vi "fp button handler_crMD.vi"(5 "dummy error input (just for timing purposes)":errorcluster) -> ()   [LabVIEW 2012]
doc: "SciScan 1.2 160622"
uses:
  <vilib>/Utility/VariantDataType/Type.ctl
  GFG/GFGallGet.vi
  GFG/GFGfpRefGet.vi
  GFG/GFG library.lvlib
  <vilib>/Utility/VariantDataType/VariantType.lvlib
panel:
  out "Source VI":string
  in  "stop":bool
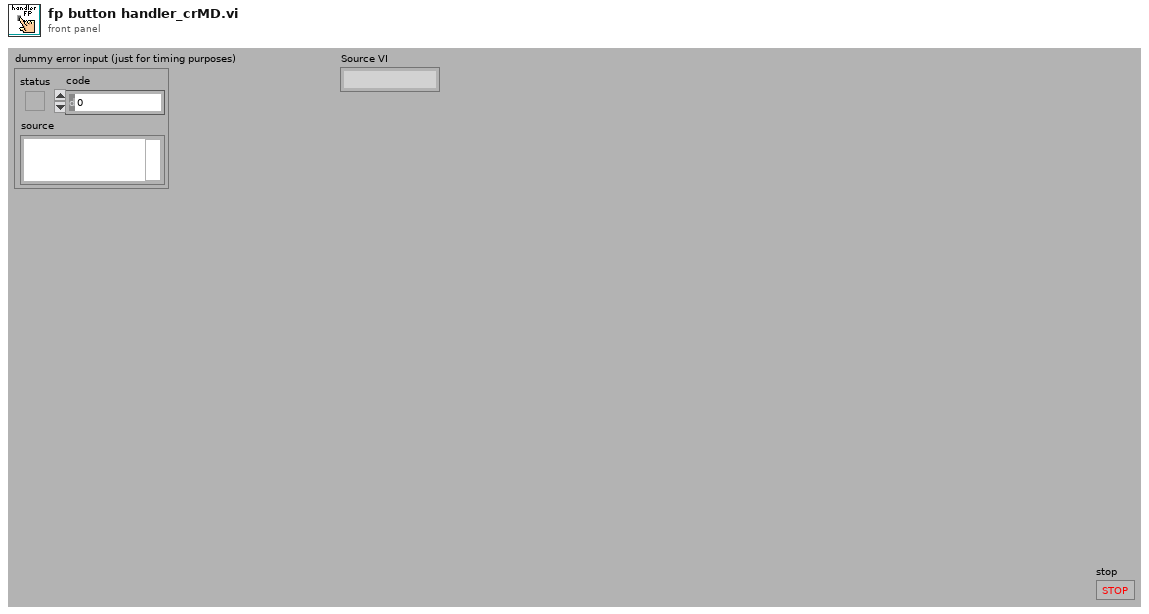
[diagram p1: front panel]
types:
  T1 = enum32{"invalid OS target", "Mac OS", "Windows 3.1", "Windows 95/NT", "Solaris 1", "Solaris 2", "HP-UX", "PowerMAX", "Linux", "Irix", "Rhapsody", "BeOS", "AIX", "OSF1", "VxWorks", "PharLap", "Carbon", "RTX", "Windows x64", "Linux x64"}
  T2 = typedef "VariantType.lvlib/Type.ctl" = enum8{"Invalid Type", "Void", "I8", "I16", "I32", "I64", "U8", "U16", "U32", "U64", "Single Float", "Double Float", "Extended Float", "Single Complex", "Double Complex", "Extended Complex", "Enum U8", "Enum U16", "Enum U32", "Enum U64", "Single Float With Unit", "Double Float With Unit", "Extended Float With Unit", "Single Complex with Unit", "Double Complex with Unit", "Extended Complex with Unit", "Boolean", "String", "Path", "Picture", "Tag", "Array", "Cluster", "Variant", "LV Variant", "Waveform", "Timestamp", "Digital Waveform", "Digital Data", "ExpressData", "Refnum", "External Data", "VI", "Poly VI", "LabVIEW Class Instance", "Fixed Point"}
  T3 = cluster{"Variable Name Out":string, "Data Type Out":T2, "Variant Out":variant}[]
  T4 = cluster{"WaveformChartRef":refnum<vi>, "DigitalRef":refnum<vi>, "ArrayRef":refnum<vi>, "TabControlRef":refnum<vi>, "EnumRef":refnum<vi>, "RingRef":refnum<vi>, "BooleanRef":refnum<vi>, "KnobRef":refnum<vi>, "SlideRef":refnum<vi>, "PathRef":refnum<vi>, "StringRef":refnum<vi>, "ComboBox":refnum<vi>, "WaveformGraphRef":refnum<vi>}
  T5 = enum8{"Enabled", "Disabled", "Disabled and Grayed Out"}
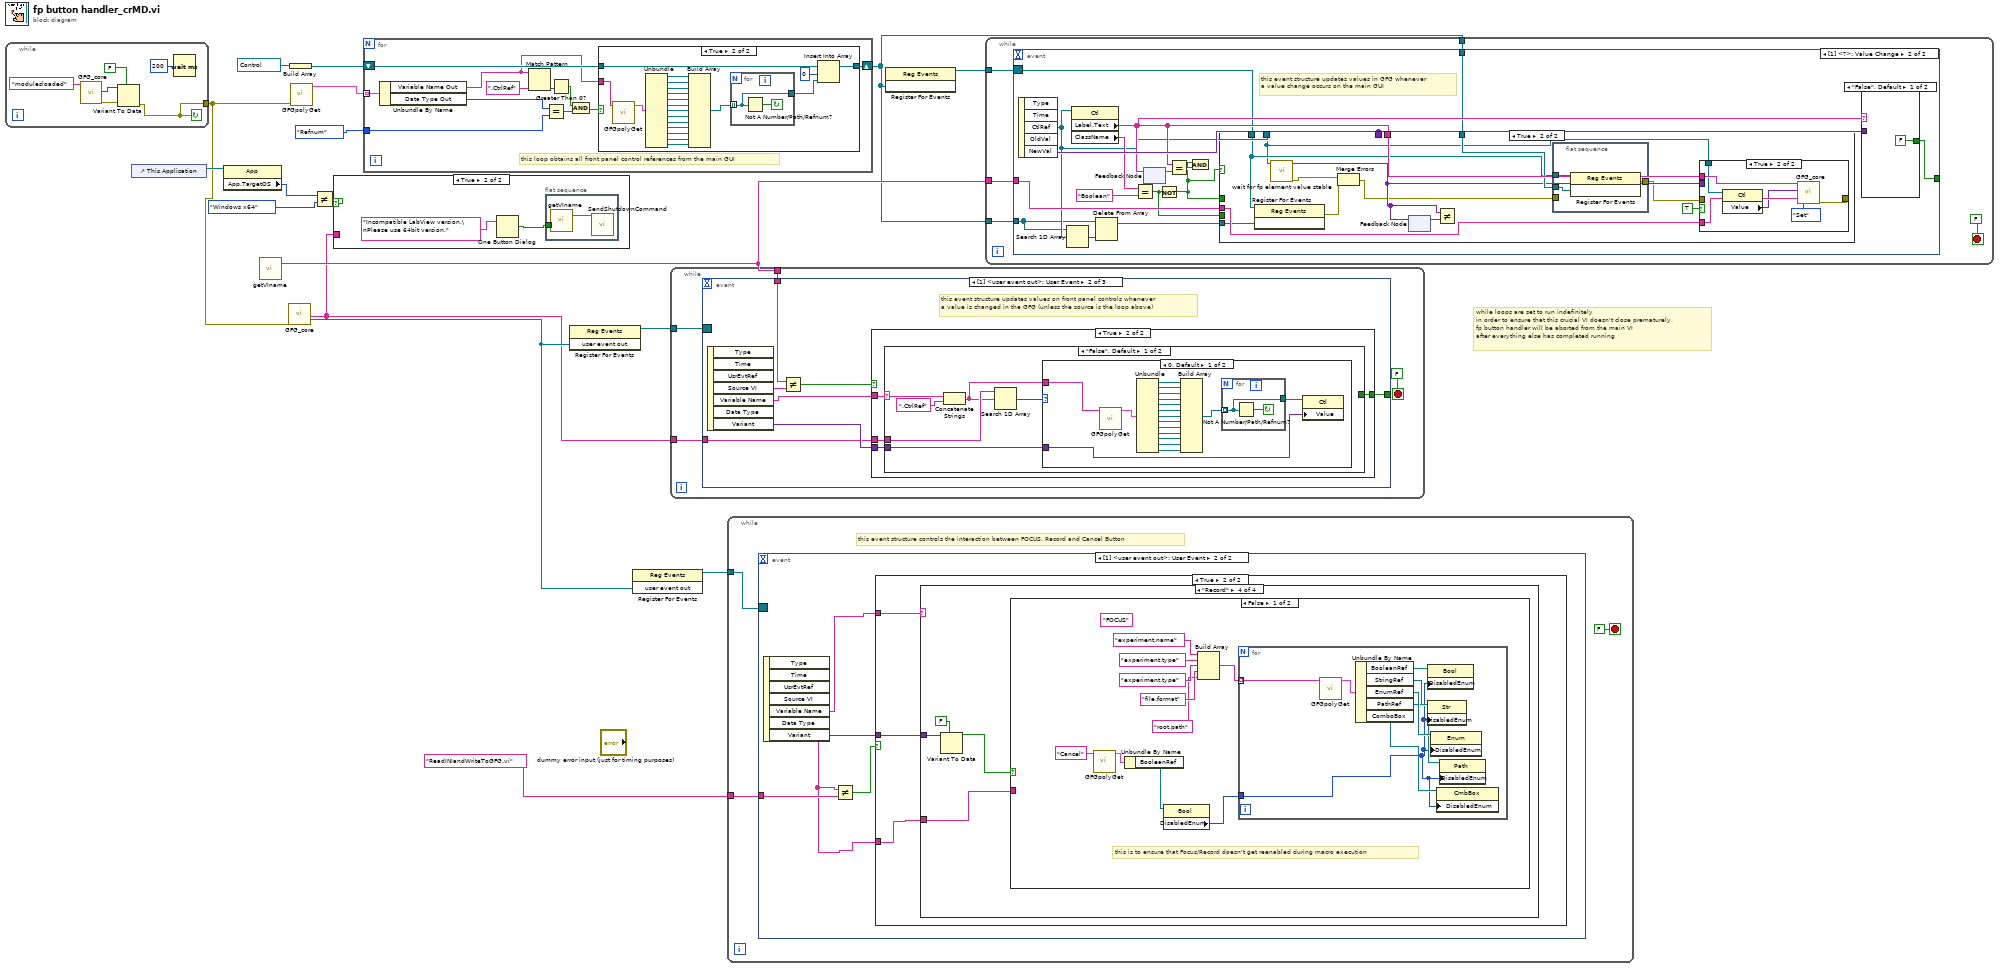
[diagram p0: block diagram]
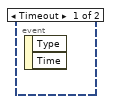
[diagram p3: hidden frame]
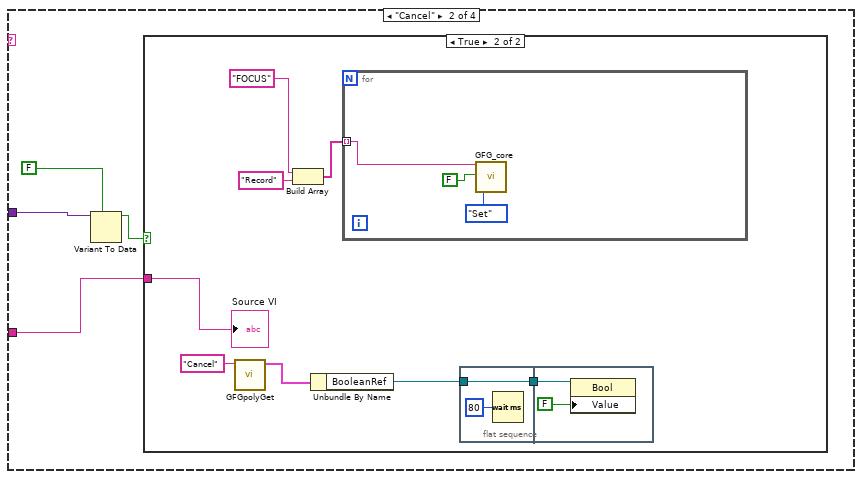
[diagram p6: hidden frame]
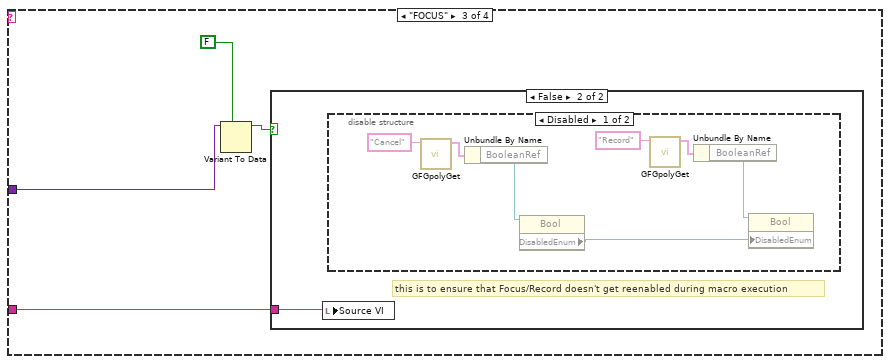
[diagram p8: hidden frame]
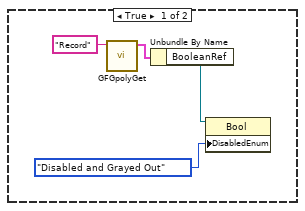
[diagram p9: hidden frame]
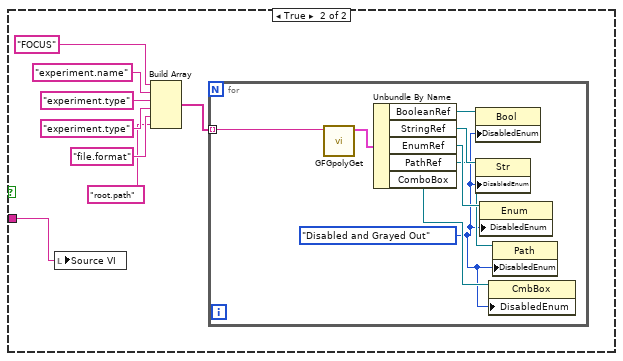
[diagram p11: hidden frame]
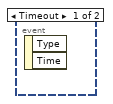
[diagram p12: hidden frame]
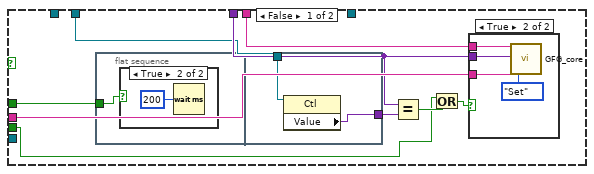
[diagram p13: hidden frame]
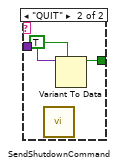
[diagram p17: hidden frame]
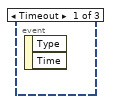
[diagram p19: hidden frame]
diagram:
  # "while loops are set to run indefinitely\nin order to ensure that this crucial VI doesn't close prematurely.\nfp button handler will be aborted from the main VI \nafter everything else has completed running"
  n1 = while {
    tunnel: [w18] -> w2
    stop <- w18 continue-if-true
    n2 = call "GFG_core.vi"("Variable Name in"="modulesloaded") -> ("Variant Out"=w19:variant, "error out"=w21:errorcluster)  [unwired: 12 in, 5 out]
    n3 = Variant To Data(error in=w21, type=FALSE, Variant=w19) -> (error out=w18:errorcluster)  [unwired: 1 out]
    n4 = Wait (ms)(milliseconds to wait=u32 200) -> ()  [unwired: 1 out]
  }
  n5 = control-ref of="This Application"() -> (w7:refnum<vi>)
  n6 = property class="App"(reference=w7) -> ("App.TargetOS"=w6:T1)  [unwired: 1 in, 2 out]
  n7 = call "getVIname.vi"() -> ("VI name"=w11:string)  [unwired: 19 in]
  n8 = call "GFG_core.vi"("error in (no error)"=w2) -> ("All Variable Names Out"=w3:string[], "user event out"=w9:refnum<user-event>)  [unwired: 12 in, 5 out]
  n9 = Build Array(refnum<vi> refnum ("DigitalRef")) -> (w14:refnum<vi>[])
  n10 = call-poly "GFGpolyGet.vi"("error in (no error)"=w2) -> ("Array of Clusters of Variables"=w16:T3)  [unwired: 9 in, 1 out]
  n11 = Not Equal?(x=w6, y=T1."Windows x64" ("Application:Target:Operating System")) -> (x != y?=w4:bool)
  n12 = case shown="True" w4 {
    tunnel: w3 -> [_ _]
    frame False {
    }
    frame True {
      n13 = One Button Dialog(message="Incompatible LabView version.\nPlease use 64bit version." ("source")) -> (true=w24:bool)  [unwired: 1 in]
      n14 = flat-sequence {
        tunnel: w24 -> [_]
        frame #0 {
          n15 = call "getVIname.vi"() -> ("VI name"=w26:string)  [unwired: 19 in]
          n16 = call "SendShutdownCommand.vi"("Source VI"=w26) -> ()  [unwired: 11 in]
        }
      }
    }
  }
  n17 = for {
    tunnel: w16 -> [w37] mode=indexing
    tunnel: Type."Refnum" ("Data Type Out") -> [w35]
    shift-right: [w33] -> w1
    shift-left: w14 -> [w34]
    # "this loop obtains all front panel control references from the main GUI"
    n18 = Unbundle By Name(w37) -> ("Variable Name Out"=w27:string, "Data Type Out"=w36:T2)
    n19 = Match Pattern(string=w27, regular expression=".CtrlRef" ("string")) -> (offset past match=w31:i32)  [unwired: 1 in, 3 out]
    n20 = Equal?(x=w36, y=w35) -> (x = y?=w28:bool)
    n21 = Greater Than 0?(x=w31) -> (x > 0?=w29:bool)
    n22 = And(x=w29, y=w28) -> (x .and. y?=w30:bool)
    n23 = case shown="True" w30 {
      tunnel: w34 -> [w38 w44]
      tunnel: [w38 w43] -> w33
      tunnel: w27 -> [_ w41]
      frame False {
      }
      frame True {
        n24 = call-poly "GFGpolyGet.vi"("Variable Name in"=w41) -> ("output cluster"=w46:T4)  [unwired: 9 in, 1 out]
        n25 = Unbundle(w46) -> ("WaveformChartRef"=w47:refnum<vi>, "DigitalRef"=w48:refnum<vi>, "ArrayRef"=w49:refnum<vi>, "TabControlRef"=w50:refnum<vi>, "EnumRef"=w51:refnum<vi>, "RingRef"=w52:refnum<vi>, "BooleanRef"=w53:refnum<vi>, "KnobRef"=w54:refnum<vi>, "SlideRef"=w55:refnum<vi>, "PathRef"=w56:refnum<vi>, "StringRef"=w57:refnum<vi>, "ComboBox"=w40:refnum<vi>, "WaveformGraphRef"=w39:refnum<vi>)
        n26 = Build Array(w47, w48, w49, w50, w51, w52, w53, w54, w55, w56, w57, w40, w39) -> (w58:refnum<vi>[])
        n27 = for {
          tunnel: w58 -> [w59] mode=indexing
          tunnel: [w59] -> w45
          stop <- w60 continue-if-true
          n28 = Not A Number/Path/Refnum?(number/path/refnum=w59) -> (NaN/Path/Refnum?=w60:bool)
        }
        n29 = Insert Into Array(array=w44, index=0, new element=w45) -> (w43:refnum<vi>[])
      }
    }
  }
  n30 = register-events(w9) -> (reference out=w17:refnum<event-registration>)  [unwired: 2 in, 1 out]
  n31 = register-events(w9) -> (reference out=w12:refnum<event-registration>)  [unwired: 2 in, 1 out]
  n32 = while {
    tunnel: w17 -> [w64]
    tunnel: w3 -> [w63]
    tunnel: w11 -> [w62]
    stop <- FALSE stop-if-true
    n33 = event shown="[1] <user event out>: User Event" {
      selector: w64 -> [_ _ _]
      dyn-events: _ -> [_ _ _]
      timeout: _ -> [_ _ _]
      tunnel: [_ w70 _] -> _
      tunnel: w63 -> [_ w69 _]
      tunnel: w62 -> [_ w68 _]
      event Timeout {
        n34 = event-data() -> ()  [unwired: 1 in, 2 out]
      }
      event User Event {
        # "this event structure updates values on front panel controls whenever\na value is changed in the GFG (unless the source is the loop above)"
        n35 = event-data() -> ("Source VI"=w65:string, "Variable Name"=w66:string, "Variant"=w71:variant)  [unwired: 1 in, 4 out]
        n36 = Not Equal?(x=w68, y=w65) -> (x != y?=w67:bool)
        n37 = case shown="True" w67 {
          tunnel: w66 -> [_ w75]
          tunnel: w71 -> [_ w74]
          tunnel: [_ w73] -> w70
          tunnel: w69 -> [_ w72]
          frame False {
          }
          frame True {
            n38 = case shown="\"False\", Default" w75 {
              selector: w75 -> [w80 _]
              tunnel: w74 -> [w76 w104]
              tunnel: [_ w102] -> w73
              tunnel: w72 -> [w79 _]
              frame "False", Default {
                n39 = Concatenate Strings(w80, ".CtrlRef" ("string")) -> (w77:string)
                n40 = Search 1D Array(1D array=w79, element=w77) -> (index of element=w78:i32)  [unwired: 1 in]
                n41 = case shown="0, Default" w78 {
                  tunnel: w77 -> [w99 _]
                  tunnel: w76 -> [w84 _]
                  frame 0, Default {
                    n42 = call-poly "GFGpolyGet.vi"("Variable Name in"=w99) -> ("output cluster"=w98:T4)  [unwired: 9 in, 1 out]
                    n43 = Unbundle(w98) -> ("WaveformChartRef"=w97:refnum<vi>, "DigitalRef"=w96:refnum<vi>, "ArrayRef"=w95:refnum<vi>, "TabControlRef"=w94:refnum<vi>, "EnumRef"=w93:refnum<vi>, "RingRef"=w92:refnum<vi>, "BooleanRef"=w91:refnum<vi>, "KnobRef"=w90:refnum<vi>, "SlideRef"=w89:refnum<vi>, "PathRef"=w88:refnum<vi>, "StringRef"=w87:refnum<vi>, "ComboBox"=w83:refnum<vi>, "WaveformGraphRef"=w82:refnum<vi>)
                    n44 = Build Array(w97, w96, w95, w94, w93, w92, w91, w90, w89, w88, w87, w83, w82) -> (w86:refnum<vi>[])
                    n45 = for {
                      tunnel: w86 -> [w100] mode=indexing
                      tunnel: [w100] -> w85
                      stop <- w101 continue-if-true
                      n46 = Not A Number/Path/Refnum?(number/path/refnum=w100) -> (NaN/Path/Refnum?=w101:bool)
                    }
                    n47 = property class="Ctl"(reference=w85, "Value"=w84) -> ()  [unwired: 1 in, 2 out]
                  }
                  frame -1 {
                  }
                }
              }
              frame "shutdown" {
                n48 = Variant To Data(type=TRUE ("want seconds? (F)"), Variant=w104) -> (data=w102:bool)  [unwired: 1 in, 1 out]
              }
            }
          }
        }
      }
      event "stop": Value Change {
        n49 = event-data() -> ()  [unwired: 1 in, 5 out]
        n50 = call "getVIname.vi"() -> ("VI name"=w105:string)  [unwired: 19 in]
        n51 = call "SendShutdownCommand.vi"("Source VI"=w105) -> ()  [unwired: 11 in]
      }
    }
  }
  n52 = while {
    tunnel: w12 -> [w108]
    tunnel: "ReadINIandWriteToGFG.vi" ("Source VI") -> [w106]
    stop <- FALSE stop-if-true
    # "this event structure controls the interaction between FOCUS, Record and Cancel Button"
    n53 = event shown="[1] <user event out>: User Event" {
      selector: w108 -> [_ _]
      dyn-events: _ -> [_ _]
      timeout: _ -> [_ _]
      tunnel: w106 -> [_ w111]
      event Timeout {
        n54 = event-data() -> ()  [unwired: 1 in, 2 out]
      }
      event User Event {
        n55 = event-data() -> ("Source VI"=w109:string, "Variable Name"=w113:string, "Variant"=w112:variant)  [unwired: 1 in, 4 out]
        n56 = Not Equal?(x=w109, y=w111) -> (x != y?=w110:bool)
        n57 = case shown="True" w110 {
          tunnel: w113 -> [_ w116]
          tunnel: w112 -> [_ w115]
          tunnel: w109 -> [_ w114]
          frame False {
          }
          frame True {
            n58 = case shown="\"Record\"" w116 {
              tunnel: w115 -> [_ w120 w138 w155]
              tunnel: w114 -> [_ w117 w136 w152]
              frame "False", Default {
              }
              frame "Cancel" {
                n59 = Variant To Data(type=FALSE, Variant=w120) -> (data=w118:bool)  [unwired: 1 in, 1 out]
                n60 = case shown="True" w118 {
                  tunnel: w117 -> [_ w124]
                  frame False {
                  }
                  frame True {
                    n61 = call-poly "GFGpolyGet.vi"("Variable Name in"="Cancel") -> ("output cluster"=w126:T4)  [unwired: 9 in, 1 out]
                    n62 = Build Array("FOCUS" ("Variable Name in"), "Record" ("element")) -> (w121:string[])
                    n63 = Unbundle By Name(w126) -> ("BooleanRef"=w125:refnum<vi>)
                    n64 = for {
                      tunnel: w121 -> [w130] mode=indexing
                      n65 = call "GFG_core.vi"("Variable Name in"=w130, "Variant in"=FALSE, "Action"=enum16{"Init", "Set", "Get"}."Set") -> ()  [unwired: 10 in, 7 out]
                    }
                    n66 = flat-sequence {
                      tunnel: w125 -> [w133]
                      tunnel: [w133] -> w128
                      tunnel: w128 -> [w135]
                      frame #0 {
                        n67 = Wait (ms)(milliseconds to wait=u32 80) -> ()  [unwired: 1 out]
                      }
                      frame #1 {
                        n68 = property class="Bool"(reference=w135, "Value"=FALSE) -> ()  [unwired: 1 in, 2 out]
                      }
                    }
                    "Source VI" <- w124
                  }
                }
              }
              frame "FOCUS" {
                n69 = Variant To Data(type=FALSE ("NewVal"), Variant=w138) -> (data=w137:bool)  [unwired: 1 in, 1 out]
                n70 = case shown="False" w137 {
                  tunnel: w136 -> [_ w144]
                  frame True {
                    n71 = call-poly "GFGpolyGet.vi"("Variable Name in"="Record") -> ("output cluster"=w141:T4)  [unwired: 9 in, 1 out]
                    n72 = Unbundle By Name(w141) -> ("BooleanRef"=w140:refnum<vi>)
                    n73 = property class="Bool"(reference=w140, "DisabledEnum"=T5."Disabled and Grayed Out" ("Disabled")) -> ()  [unwired: 1 in, 2 out]
                  }
                  frame False {
                    # "this is to ensure that Focus/Record doesn't get reenabled during macro execution"
                    n74 = local write "Source VI"(w144) -> ()
                    n75 = disable-structure shown="Disabled" {
                      frame Disabled {
                        n76 = call-poly "GFGpolyGet.vi"("Variable Name in"="Cancel") -> ("output cluster"=w147:T4)  [unwired: 9 in, 1 out]
                        n77 = Unbundle By Name(w147) -> ("BooleanRef"=w148:refnum<vi>)
                        n78 = property class="Bool"(reference=w148) -> ("DisabledEnum"=w145:T5)  [unwired: 1 in, 2 out]
                        n79 = call-poly "GFGpolyGet.vi"("Variable Name in"="Record") -> ("output cluster"=w150:T4)  [unwired: 9 in, 1 out]
                        n80 = Unbundle By Name(w150) -> ("BooleanRef"=w149:refnum<vi>)
                        n81 = property class="Bool"(reference=w149, "DisabledEnum"=w145) -> ()  [unwired: 1 in, 2 out]
                      }
                      frame Enabled {
                      }
                    }
                  }
                }
              }
              frame "Record" {
                n82 = Variant To Data(type=FALSE ("NewVal"), Variant=w155) -> (data=w153:bool)  [unwired: 1 in, 1 out]
                n83 = case shown="False" w153 {
                  tunnel: w152 -> [_ w174]
                  frame False {
                    (unwired) "FOCUS" ("Variable Name in")
                    # "this is to ensure that Focus/Record doesn't get reenabled during macro execution"
                    n84 = call-poly "GFGpolyGet.vi"("Variable Name in"="Cancel") -> ("output cluster"=w158:T4)  [unwired: 9 in, 1 out]
                    n85 = Unbundle By Name(w158) -> ("BooleanRef"=w159:refnum<vi>)
                    n86 = property class="Bool"(reference=w159) -> ("DisabledEnum"=w156:T5)  [unwired: 1 in, 2 out]
                    n87 = Build Array("experiment.name" ("element"), "experiment.type" ("element"), "experiment.type" ("element"), "file.format" ("element"), "root.path" ("element")) -> (w161:string[])
                    n88 = for {
                      tunnel: w161 -> [w171] mode=indexing
                      tunnel: w156 -> [w166]
                      n89 = call-poly "GFGpolyGet.vi"("Variable Name in"=w171) -> ("output cluster"=w173:T4)  [unwired: 9 in, 1 out]
                      n90 = Unbundle By Name(w173) -> ("BooleanRef"=w172:refnum<vi>, "StringRef"=w170:refnum<vi>, "EnumRef"=w169:refnum<vi>, "PathRef"=w168:refnum<vi>, "ComboBox"=w167:refnum<vi>)
                      n91 = property class="Bool"(reference=w172, "DisabledEnum"=w166) -> ()  [unwired: 1 in, 2 out]
                      n92 = property class="Str"(reference=w170, "DisabledEnum"=w166) -> ()  [unwired: 1 in, 2 out]
                      n93 = property class="Enum"(reference=w169, "DisabledEnum"=w166) -> ()  [unwired: 1 in, 2 out]
                      n94 = property class="CmbBox"(reference=w167, "DisabledEnum"=w166) -> ()  [unwired: 1 in, 2 out]
                      n95 = property class="Path"(reference=w168, "DisabledEnum"=w166) -> ()  [unwired: 1 in, 2 out]
                    }
                  }
                  frame True {
                    n96 = local write "Source VI"(w174) -> ()
                    n97 = Build Array("FOCUS" ("Variable Name in"), "experiment.name" ("element"), "experiment.type" ("element"), "experiment.type" ("element"), "file.format" ("element"), "root.path" ("element")) -> (w176:string[])
                    n98 = for {
                      tunnel: w176 -> [w187] mode=indexing
                      w182 = T5."Disabled and Grayed Out" ("Disabled")
                      n99 = call-poly "GFGpolyGet.vi"("Variable Name in"=w187) -> ("output cluster"=w189:T4)  [unwired: 9 in, 1 out]
                      n100 = Unbundle By Name(w189) -> ("BooleanRef"=w188:refnum<vi>, "StringRef"=w186:refnum<vi>, "EnumRef"=w185:refnum<vi>, "PathRef"=w184:refnum<vi>, "ComboBox"=w183:refnum<vi>)
                      n101 = property class="Bool"(reference=w188, "DisabledEnum"=w182) -> ()  [unwired: 1 in, 2 out]
                      n102 = property class="Str"(reference=w186, "DisabledEnum"=w182) -> ()  [unwired: 1 in, 2 out]
                      n103 = property class="Enum"(reference=w185, "DisabledEnum"=w182) -> ()  [unwired: 1 in, 2 out]
                      n104 = property class="CmbBox"(reference=w183, "DisabledEnum"=w182) -> ()  [unwired: 1 in, 2 out]
                      n105 = property class="Path"(reference=w184, "DisabledEnum"=w182) -> ()  [unwired: 1 in, 2 out]
                    }
                  }
                }
              }
            }
          }
        }
      }
    }
  }
  n106 = register-events(w1) -> (reference out=w13:refnum<event-registration>)  [unwired: 2 in, 1 out]
  n107 = while {
    tunnel: w13 -> [w194]
    tunnel: w11 -> [w193]
    tunnel: w1 -> [w191]
    tunnel: w1 -> [w190]
    stop <- FALSE stop-if-true
    n108 = event shown="[1] <?>: Value Change" {
      selector: w194 -> [_ w205]
      dyn-events: _ -> [_ _]
      timeout: _ -> [_ _]
      tunnel: w193 -> [_ w210]
      tunnel: [_ w209] -> _
      tunnel: w191 -> [_ w204]
      tunnel: w190 -> [_ w197]
      event Timeout {
        n109 = event-data() -> ()  [unwired: 1 in, 2 out]
      }
      event Value Change {
        # "this event structure updates values in GFG whenever\na value change occurs on the main GUI"
        n110 = event-data() -> ("CtlRef"=w199:refnum<vi>, "NewVal"=w208:variant)  [unwired: 1 in, 3 out]
        n111 = Search 1D Array(1D array=w197, element=w199) -> (index of element=w198:i32)  [unwired: 1 in]
        n112 = property class="Ctl"(reference=w199) -> ("Label.Text"=w207:string, "ClassName"=w202:string)  [unwired: 1 in, 2 out]
        n113 = Delete From Array(array=w197, index=w198) -> (array with subset deleted=w196:refnum<vi>[])  [unwired: 1 in, 1 out]
        n114 = Equal?(x=w202, y="Boolean" ("Class Name")) -> (x = y?=w200:bool)
        n115 = feedback-in #1(w207) -> ()
        n116 = feedback #1() -> (w206:string)  [unwired: 1 in]
        n117 = Not(x=w200) -> (.not. x?=w195:bool)
        n118 = Equal?(x=w207, y=w206) -> (x = y?=w203:bool)
        n119 = And(x=w195, y=w203) -> ()  [unwired: 1 out]
        n120 = case shown="True" w195 {
          tunnel: w210 -> [w219 w238]
          tunnel: w207 -> [w218 w240]
          tunnel: w208 -> [w217 _]
          tunnel: w205 -> [_ w233]
          tunnel: w199 -> [w214 w229]
          tunnel: w204 -> [_ w239]
          tunnel: w195 -> [w213 _]
          tunnel: w200 -> [w211 _]
          tunnel: w196 -> [_ w234]
          frame False {
            n121 = flat-sequence {
              tunnel: w213 -> [w224]
              tunnel: [w227] -> w216
              tunnel: w214 -> [w226]
              frame #0 {
                n122 = case shown="True" w224 {
                  frame False {
                  }
                  frame True {
                    n123 = Wait (ms)(milliseconds to wait=u32 200) -> ()  [unwired: 1 out]
                  }
                }
              }
              frame #1 {
                n124 = property class="Ctl"(reference=w226) -> ("Value"=w227:variant)  [unwired: 1 in, 2 out]
              }
            }
            n125 = Equal?(x=w217, y=w216) -> (x = y?=w215:bool)
            n126 = Or(x=w211, y=w215) -> (x .or. y?=w212:bool)
            n127 = case shown="True" w212 {
              tunnel: w219 -> [_ w222]
              tunnel: w218 -> [_ w221]
              tunnel: w217 -> [_ w220]
              frame False {
              }
              frame True {
                n128 = call "GFG_core.vi"("Variable Name in"=w221, "Variant in"=w220, "Source VI"=w222, "Action"=enum16{"Init", "Set", "Get"}."Set") -> ()  [unwired: 9 in, 7 out]
              }
            }
          }
          frame True {
            n129 = register-events(reference=w233, w234) -> (error out=w235:errorcluster)  [unwired: 1 in, 1 out]
            n130 = call "wait for fp element value stable.vi"("CtlRef"=w229) -> ("error out"=w232:errorcluster, "Value"=w236:variant)  [unwired: 9 in]
            n131 = Merge Errors(w232, w235) -> (w231:errorcluster)
            n132 = feedback #2() -> (w237:variant)  [unwired: 1 in]
            n133 = feedback-in #2(w236) -> ()
            n134 = Not Equal?(x=w236, y=w237) -> ()  [unwired: 1 out]
            n135 = flat-sequence {
              tunnel: w233 -> [w243]
              tunnel: w239 -> [w242]
              tunnel: w231 -> [_]
              tunnel: [w241] -> w230
              frame #0 {
                n136 = register-events(reference=w243, w242) -> (error out=w241:errorcluster)  [unwired: 1 in, 1 out]
              }
            }
            n137 = case shown="True" TRUE {
              tunnel: w240 -> [_ w249]
              tunnel: w236 -> [_ _]
              tunnel: [w244 w248] -> _
              tunnel: w238 -> [_ w247]
              tunnel: w230 -> [w244 _]
              tunnel: w229 -> [_ w246]
              frame False {
              }
              frame True {
                n138 = property class="Ctl"(reference=w246) -> ("Value"=w245:variant)  [unwired: 1 in, 2 out]
                n139 = call "GFG_core.vi"("Variable Name in"=w249, "Variant in"=w245, "Source VI"=w247, "Action"=enum16{"Init", "Set", "Get"}."Set") -> ("error out"=w248:errorcluster)  [unwired: 9 in, 6 out]
              }
            }
          }
        }
        n140 = case shown="\"False\", Default" w207 {
          tunnel: w208 -> [_ w254]
          tunnel: [FALSE w252] -> w209
          frame "False", Default {
          }
          frame "QUIT" {
            n141 = call "SendShutdownCommand.vi"() -> ()  [unwired: 12 in]
            n142 = Variant To Data(type=TRUE, Variant=w254) -> (data=w252:bool)  [unwired: 1 in, 1 out]
          }
        }
      }
    }
  }
